vi "RowAndColumnToMap.vi"(10 "Column":i32, 11 "Row":i32) -> (3 "map":map{string, i32}(c390))   [LabVIEW 2020]
doc: "Converts an input of row + Column to a map output for piece selection"
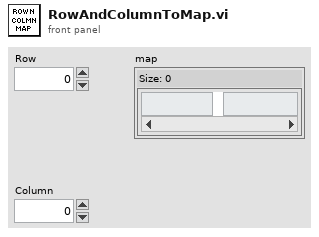
[diagram p1: front panel]
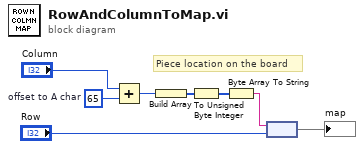
[diagram p0: block diagram]
diagram:
  w1 = 65  # offset to A char
  # "Piece location on the board"
  n1 = Add(x="Column", y=w1) -> (x+y=w2:i32)
  n2 = Build Array(w2) -> (w4:i32[])
  n3 = To Unsigned Byte Integer(number=w4) -> (unsigned 8bit integer=w5:u8[])
  n4 = Byte Array To String(unsigned byte array=w5) -> (string=w3:string)
  n5 = node(w3, "Row") -> (→"map":map{string, i32})
